vi "MGSE Log.vi"(7 "Log Ref":refnum<vi>, 8 "error in (no error)":errorcluster, 10 "Action":T1, 11 "Log Message":string) -> (0 "error out":errorcluster, 3 "Log":string)   [LabVIEW 2018]
uses:
  MGSE enum Log Action.ctl
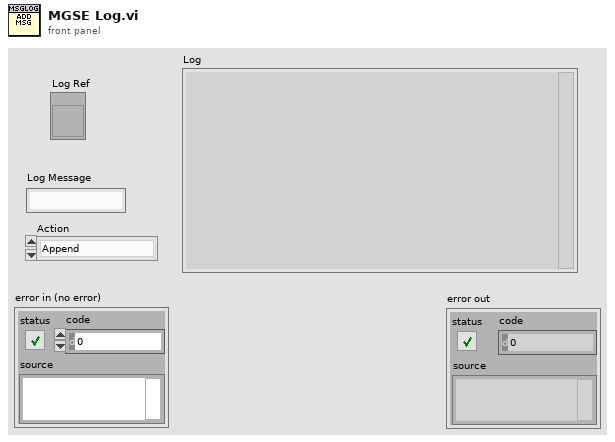
[diagram p1: front panel]
types:
  T1 = typedef "MGSE enum Log Action.ctl" = enum16{"Append", "Clear", "Retrieve"}
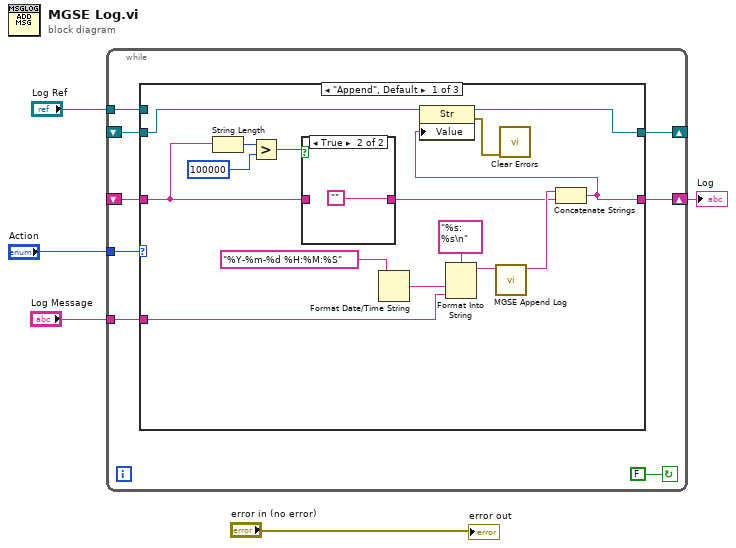
[diagram p0: block diagram]
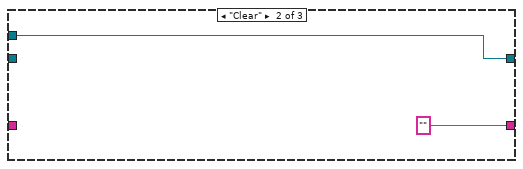
[diagram p3: hidden frame]
diagram:
  n1 = while {
    tunnel: "Action" -> [w13]
    shift-right: [w12] -> w3
    shift-left: _ -> [w11]
    tunnel: "Log Message" -> [w10]
    shift-right: [w8] -> _
    shift-left: _ -> [w6]
    tunnel: "Log Ref" -> [w7]
    stop <- FALSE continue-if-true
    n2 = case shown="\"Append\", Default" w13 {
      tunnel: [w17 "" w34] -> w12
      tunnel: w11 -> [w21 _ w34]
      tunnel: w10 -> [w25 _ _]
      tunnel: [w16 w31 w33] -> w8
      tunnel: w7 -> [_ w31 _]
      tunnel: w6 -> [w14 _ w33]
      frame "Append", Default {
        n3 = String Length(string=w21) -> (length=w24:i32)
        n4 = Greater?(x=w24, y=100000) -> (0:w22:bool)
        n5 = case shown="True" w22 {
          tunnel: w21 -> [w29 _]
          tunnel: [w29 ""] -> w18
          frame False {
          }
          frame True {
          }
        }
        n6 = Format Date/Time String(time format string (%c)="%Y-%m-%d %H:%M:%S") -> (date/time string=w26:string)  [unwired: 2 in]
        n7 = Format Into String(format string="%s: %s\n", w26, w25) -> (resulting string=w20:string)  [unwired: 2 in, 1 out]
        n8 = call "MGSE Append Log.vi"("Log Line"=w20) -> ("log dup"=w19:string)  [unwired: 10 in]
        n9 = Concatenate Strings(w19, w18) -> (w17:string)
        n10 = property class="Str"(reference=w14, "Value"=w17) -> (reference out=w16:refnum<vi>, error out=w15:errorcluster)  [unwired: 1 in]
        n11 = call <vilib>:"Clear Errors.vi"("error in (no error)"=w15) -> ()  [unwired: 5 in, 2 out]
      }
      frame "Clear" {
      }
      frame "Retrieve" {
      }
    }
  }
  "Log" <- w3
  "error out" <- "error in (no error)"
